vi "MTS_TCSPCBinnAndSum.vi"(7 "TCSPC Binning":i32[][](array[numeric]), 11 "TCSPC Histogram":i32[][](array[numeric])) -> (3 "Intensity Values":i32[](array[numeric]))   [LabVIEW 2013]
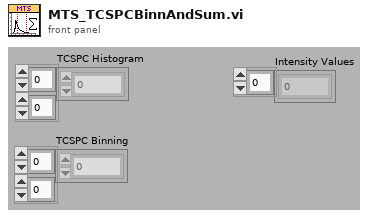
[diagram p1: front panel]
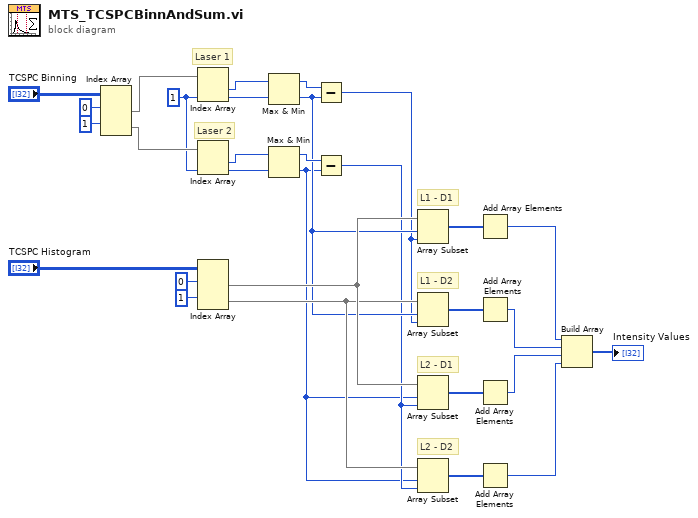
[diagram p0: block diagram]
diagram:
  w25 = 1 ("index")
  # "L2 - D2"
  # "L2 - D1"
  # "L1 - D2"
  # "L1 - D1"
  # "Laser 2"
  # "Laser 1"
  n1 = Index Array(array="TCSPC Binning", index (row) #1=0 ("index (row)"), index (row) #2=1 ("index (row)")) -> (element #1=w27:i32[], element #2=w26:i32[])  [unwired: 2 in]
  n2 = Index Array(array=w27, index #2=w25) -> (element #1=w21:i32, element #2=w20:i32)  [unwired: 1 in]
  n3 = Index Array(array=w26, index #2=w25) -> (element #1=w18:i32, element #2=w19:i32)  [unwired: 1 in]
  n4 = Index Array(array="TCSPC Histogram", index (row) #1=0 ("index (row)"), index (row) #2=1 ("index (row)")) -> (element #1=w15:i32[], element #2=w14:i32[])  [unwired: 2 in]
  n5 = Max & Min(x=w21, y=w20) -> (max(x,y)=w17:i32, min(x,y)=w13:i32)
  n6 = Max & Min(x=w18, y=w19) -> (max(x,y)=w16:i32, min(x,y)=w10:i32)
  n7 = Subtract(x=w17, y=w13) -> (x-y=w12:i32)
  n8 = Subtract(x=w16, y=w10) -> (x-y=w11:i32)
  n9 = Array Subset(array=w15, index=w13, length=w12) -> (w8:i32[])
  n10 = Array Subset(array=w14, index=w13, length=w12) -> (w5:i32[])
  n11 = Array Subset(array=w15, index=w10, length=w11) -> (w6:i32[])
  n12 = Array Subset(array=w14, index=w10, length=w11) -> (w7:i32[])
  n13 = Add Array Elements(numeric array=w8) -> (sum=w3:i32)
  n14 = Add Array Elements(numeric array=w5) -> (sum=w2:i32)
  n15 = Add Array Elements(numeric array=w6) -> (sum=w1:i32)
  n16 = Add Array Elements(numeric array=w7) -> (sum=w4:i32)
  n17 = Build Array(w3, w2, w1, w4) -> (→"Intensity Values":i32[])
